vi "InitUSB4000.vi"(1 "Int Time (usec)":i32=1000000) -> (0 "USB4000 Params":T1)   [LabVIEW 2012]
panel:
  out "Spect*":u32
  out "Number of Spectrometers":i32
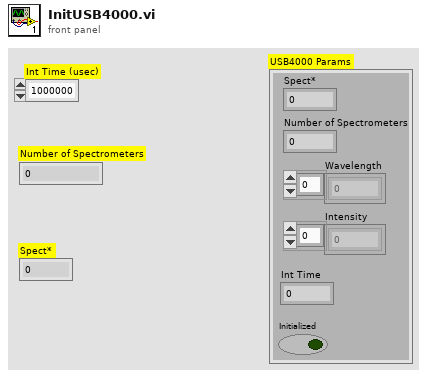
[diagram p1: front panel]
types:
  T1 = cluster{"Spect*":u32, "Number of Spectrometers":i32, "Wavelength":dbl[], "Intensity":dbl[], "Int Time":i32, "Initialized":bool}
  T2 = cluster{"Wrapper Out":u32, "Number of Spectrometers":i32, "Wavelength":dbl[], "Wavelength":dbl[], "Int Time (usec)":i32, bool}
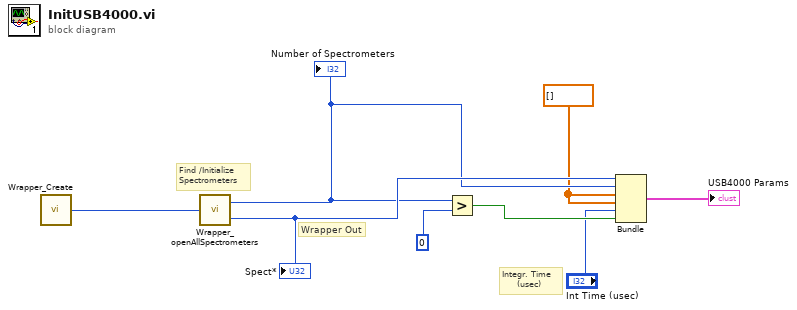
[diagram p0: block diagram]
diagram:
  w4 = dbl[] [] ("Wavelength")
  # "Integr. Time\n     (usec)"
  # "Wrapper Out"
  # "Find /Initialize\nSpectrometers"
  n1 = call "Wrapper_Create.vi"() -> ("Wrapper"=w8:u32)
  n2 = call "Wrapper_openAllSpectrometers.vi"("Wrapper In"=w8) -> ("Number of Spectrometers"=w5:i32, "Wrapper Out"=w6:u32)
  "Number of Spectrometers" <- w5
  "Spect*" <- w6
  n3 = Greater?(x=w5, y=0) -> (0:w3:bool)
  n4 = Bundle("Wrapper Out"=w6, "Number of Spectrometers"=w5, "Wavelength"=w4, "Wavelength"=w4, "Int Time (usec)"="Int Time (usec)", w3) -> (→"USB4000 Params":T2)  [unwired: 1 in]
